vi "Thermistor_Pt1000.vi"() -> ()   [LabVIEW 2025]
uses:
  <vilib>/DAQmx/read.llb/DAQmx Read (Analog DBL 1Chan 1Samp).vi
  <vilib>/DAQmx/create/channels.llb/DAQmx Create Channel (AI-Voltage-Basic).vi
  <vilib>/DAQmx/miscellaneous.llb/DAQmx Fill In Error Info.vi
panel:
  in  "ThermistorTruePt1000False":bool
  in  "Alfa":dbl
  in  "Gain Correction":dbl
  in  "Offset Correction":dbl
  in  "RT0":sgl=-10.0
  in  "V1CC":sgl=-10.0
  in  "R1":sgl=-10.0
  in  "Beta":sgl=-10.0
  out "Voltage":dbl
  out "Kelvin":bool
  out "Celsius":bool
  in  "Kelvin to Celsius":bool
  in  "Stop":bool
  in  "Real Instrument":bool
  in  "VREFN":sgl=-10.0
  in  "VREFP":sgl=10.0
  in  "Output Voltage":dbl
  out "Temperature":dbl(graph)
  in  "RESET":bool
  out "min, MAX":cluster{dbl, dbl}(graph)
  out "Average":dbl(graph)
  out "Abs Minimum":dbl
  out "Averaging Sub-Step":i32
  in  "Moving Averaging Samples":i32
  out "Iteration":i32
  out "Average":dbl
  out "Abs Maximum":dbl
  in  "ms to wait":i32
  in  "N of Iterations":i32
  out "Temperature":dbl
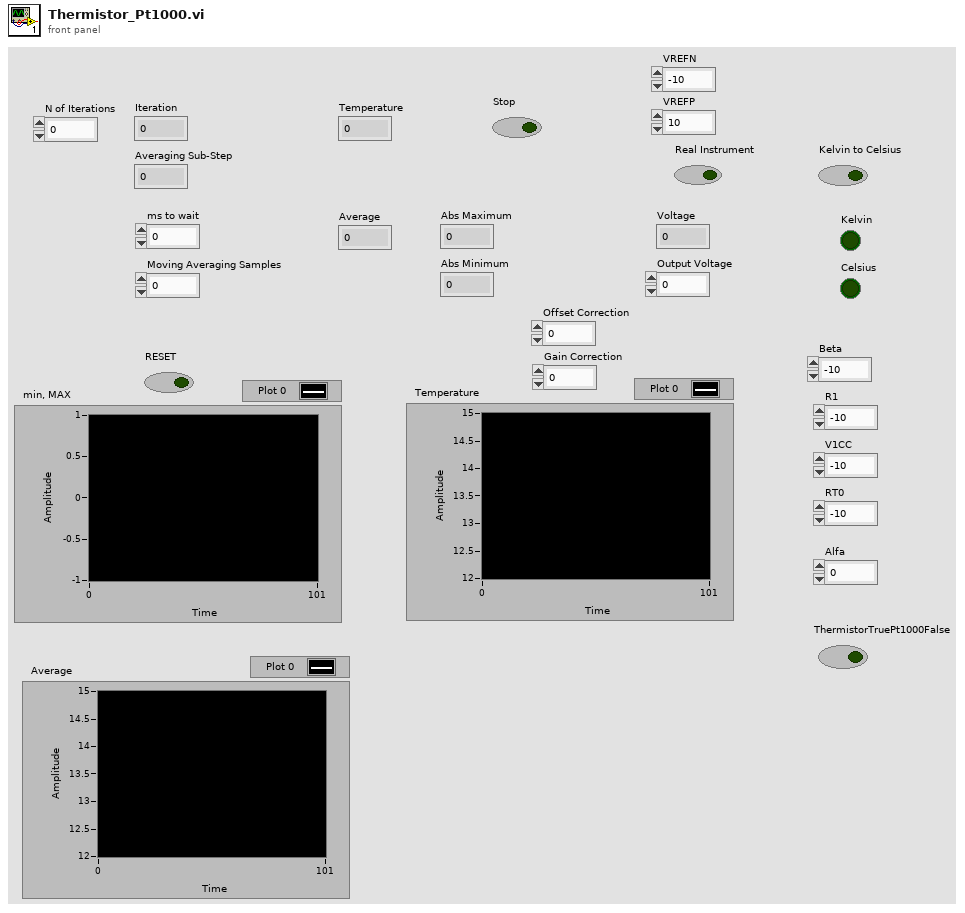
[diagram p1: front panel]
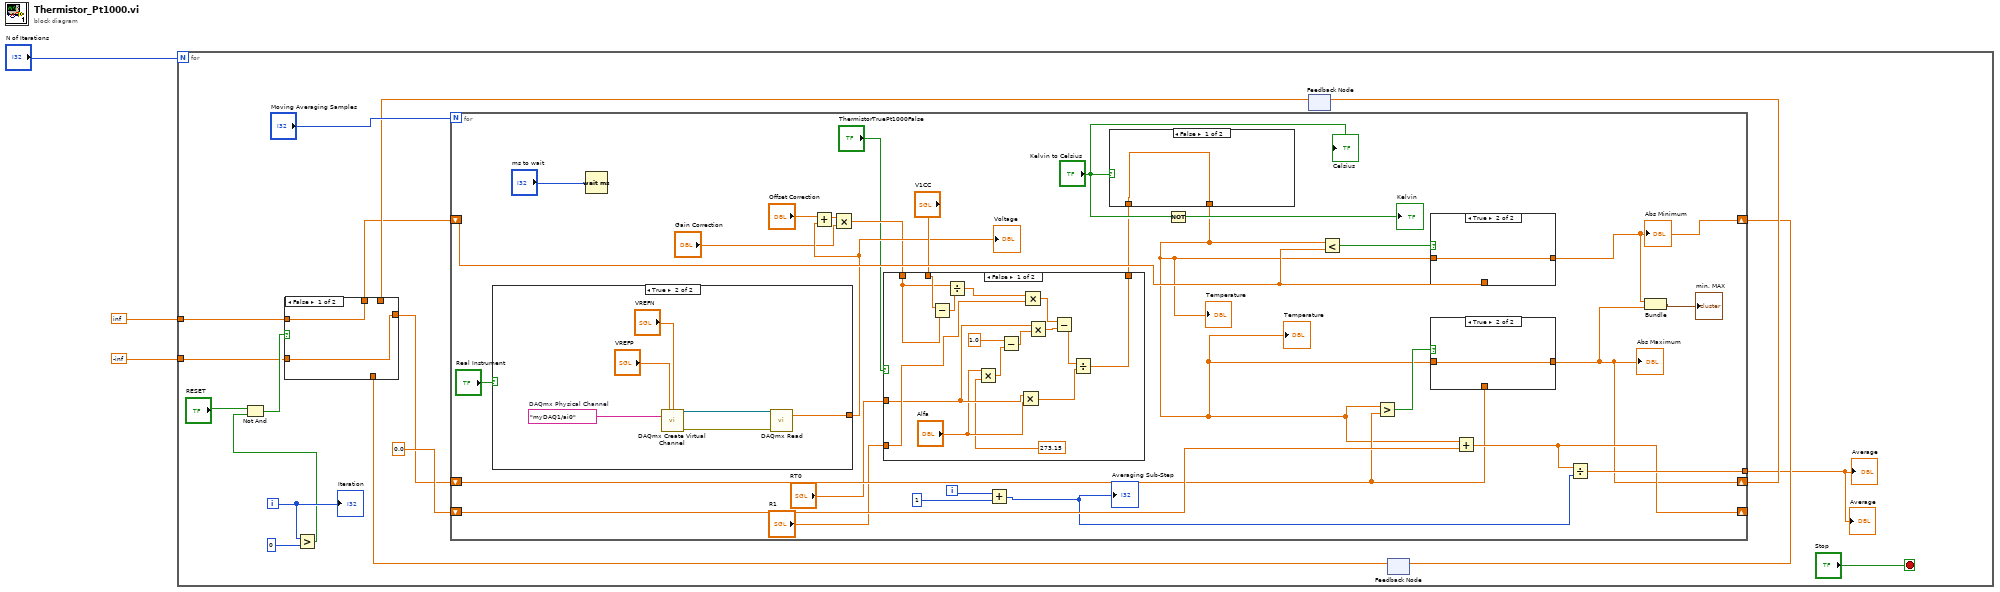
[diagram p0: block diagram]
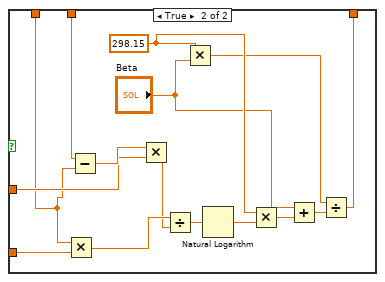
[diagram p3: hidden frame]
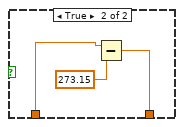
[diagram p4: hidden frame]
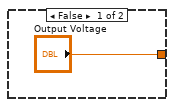
[diagram p5: hidden frame]
diagram:
  n1 = for {
    N: "N of Iterations" -> [_]
    tunnel: inf -> [w5]
    tunnel: -inf -> [w4]
    i -> [w18]
    stop <- "Stop" stop-if-true
    n2 = Greater?(x=w18, y=i8 0) -> (0:w9:bool)
    n3 = Not And(1:w9, 2:"RESET") -> (0:w8:bool)
    n4 = feedback #1() -> (w14:dbl)  [unwired: 1 in]
    n5 = feedback #2() -> (w11:dbl)  [unwired: 1 in]
    n6 = case shown="False" w8 {
      tunnel: [w21 w24] -> w16
      tunnel: w14 -> [_ w24]
      tunnel: [w22 w23] -> w13
      tunnel: w11 -> [_ w23]
      tunnel: w5 -> [w22 _]
      tunnel: w4 -> [w21 _]
      frame False {
      }
      frame True {
      }
    }
    n7 = for {
      N: "Moving Averaging Samples" -> [_]
      tunnel: [w52] -> w6
      shift-right: [w51] -> _
      shift-left: 0.0 -> [w50]
      shift-right: [w43] -> w15
      shift-left: w16 -> [w48]
      shift-right: [w44] -> w12
      shift-left: w13 -> [w45]
      i -> [w27]
      n8 = case shown="True" "Real Instrument" {
        tunnel: ["Output Voltage" w89] -> w32
        frame False {
        }
        frame True {
          w92 = tag "myDAQ1/ai0"  # DAQmx Physical Channel
          n9 = call-poly <vilib>:"DAQmx Create Virtual Channel.vi"("maximum value"="VREFP", "minimum value"="VREFN", "physical channels"=w92) -> ("task out"=w94:refnum<k21>, "error out"=w93:errorcluster)  [unwired: 11 in]
          n10 = call-poly <vilib>:"DAQmx Read.vi"("task/channels in"=w94, "error in"=w93) -> ("data"=w89:dbl)  [unwired: 11 in, 2 out]
        }
      }
      "Voltage" <- w32
      n11 = Wait (ms)(milliseconds to wait="ms to wait") -> ()  [unwired: 1 out]
      n12 = Add(x="Offset Correction", y=w32) -> (x+y=w30:dbl)
      n13 = Multiply(x=w30, y="Gain Correction") -> (x*y=w31:dbl)
      n14 = case shown="False" "ThermistorTruePt1000False" {
        tunnel: "R1" -> [w63 w83]
        tunnel: "V1CC" -> [w66 w82]
        tunnel: "RT0" -> [w58 w76]
        tunnel: [w68 w70] -> w35
        tunnel: w31 -> [w65 w69]
        frame False {
          n15 = Subtract(x=w66, y=w65) -> (x-y=w64:dbl)
          n16 = Divide(x=w65, y=w64) -> (x/y=w62:dbl)
          n17 = Multiply(x="Alfa", y=273.15) -> (x*y=w56:dbl)
          n18 = Subtract(x=1.0, y=w56) -> (x-y=w53:dbl)
          n19 = Multiply(x=w58, y="Alfa") -> (x*y=w67:dbl)
          n20 = Multiply(x=w62, y=w63) -> (x*y=w61:dbl)
          n21 = Multiply(x=w58, y=w53) -> (x*y=w59:dbl)
          n22 = Subtract(x=w61, y=w59) -> (x-y=w60:dbl)
          n23 = Divide(x=w60, y=w67) -> (x/y=w68:dbl)
        }
        frame True {
          w75 = 298.15
          n24 = Multiply(x=w69, y=w83) -> (x*y=w80:dbl)
          n25 = Subtract(x=w82, y=w69) -> (x-y=w81:dbl)
          n26 = Multiply(x=w81, y=w76) -> (x*y=w79:dbl)
          n27 = Divide(x=w80, y=w79) -> (x/y=w78:dbl)
          n28 = Multiply(x=w75, y="Beta") -> (x*y=w71:dbl)
          n29 = Natural Logarithm(1:w78) -> (0:w77:dbl)
          n30 = Multiply(x=w75, y=w77) -> (x*y=w74:dbl)
          n31 = Add(x="Beta", y=w74) -> (x+y=w72:dbl)
          n32 = Divide(x=w71, y=w72) -> (x/y=w70:dbl)
        }
      }
      n33 = Add(x=w27, y=1) -> (x+y=w28:i32)
      "Averaging Sub-Step" <- w28
      n34 = case shown="False" "Kelvin to Celsius" {
        tunnel: w35 -> [w84 w86]
        tunnel: [w84 w85] -> w34
        frame False {
        }
        frame True {
          n35 = Subtract(x=w86, y=273.15) -> (x-y=w85:dbl)
        }
      }
      "Temperature" <- w34
      "Temperature" <- w34
      n36 = Not(x="Kelvin to Celsius") -> (.not. x?=→"Kelvin":bool)
      n37 = Less?(x=w34, y=w45) -> (x < y?=w46:bool)
      n38 = Greater?(x=w34, y=w48) -> (0:w49:bool)
      n39 = case shown="True" w46 {
        tunnel: [w95 w96] -> w44
        tunnel: w34 -> [_ w96]
        tunnel: w45 -> [w95 _]
        frame False {
        }
        frame True {
        }
      }
      "Abs Minimum" <- w44
      n40 = case shown="True" w49 {
        tunnel: [w97 w98] -> w43
        tunnel: w34 -> [_ w98]
        tunnel: w48 -> [w97 _]
        frame False {
        }
        frame True {
        }
      }
      "Abs Maximum" <- w43
      n41 = Add(x=w34, y=w50) -> (x+y=w51:dbl)
      n42 = Divide(x=w51, y=w28) -> (x/y=w52:dbl)
      n43 = Bundle(w44, w43) -> (→"min, MAX":cluster{dbl, dbl})  [unwired: 1 in]
      "Celsius" <- "Kelvin to Celsius"
    }
    "Average" <- w6
    "Average" <- w6
    n44 = feedback-in #1(w15) -> ()
    n45 = feedback-in #2(w12) -> ()
    "Iteration" <- w18
  }
